vi "Auto-IR Logic.vi"(4 "Reset":bool, 6 "Upper Mag IR":T1, 7 "Rear Enter IR":T1) -> (0 "Finished":bool, 1 "Roller Output":dbl, 2 "Upper Mag IR Out":T1, 3 "Rear Enter IR Out":T1)   [LabVIEW 2011]
uses:
  <vilib>/Rock Robotics/WPI/DigitalInput/WPI_DigitalInputDevRef.ctl
  <vilib>/Rock Robotics/SystemInterfaces/DIO/FPGA_DIOChannel.ctl
  <vilib>/Rock Robotics/SystemInterfaces/Typedef/FPGA_TypedefDigitalModule.ctl
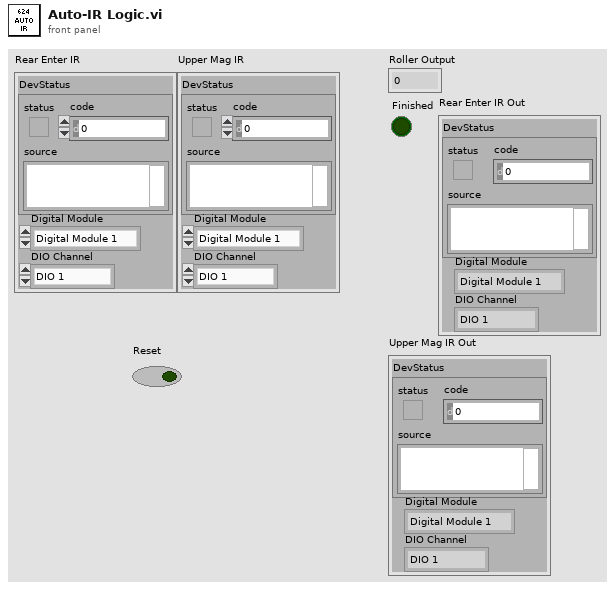
[diagram p1: front panel]
types:
  T1 = typedef "WPI_DigitalInputDevRef.ctl" = cluster{"DevStatus":errorcluster, "DIO Channel":T2, "Digital Module":T3}
  T2 = typedef "FPGA_DIOChannel.ctl" = enum8{"DIO 1", "DIO 2", "DIO 3", "DIO 4", "DIO 5", "DIO 6", "DIO 7", "DIO 8", "DIO 9", "DIO 10", "DIO 11", "DIO 12", "DIO 13", "DIO 14", "Invalid"}
  T3 = typedef "FPGA_TypedefDigitalModule.ctl" = enum16{"Digital Module 1", "Digital Module 2"}
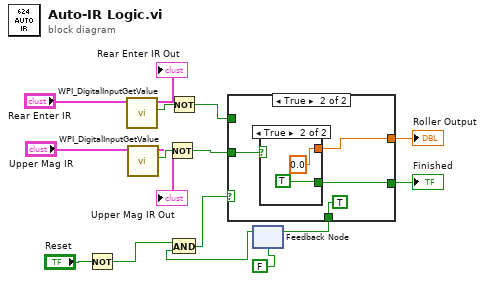
[diagram p0: block diagram]
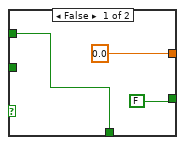
[diagram p2: hidden frame]
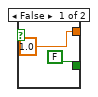
[diagram p3: hidden frame]
diagram:
  n1 = Not(x="Reset") -> (.not. x?=w5:bool)
  n2 = call <vilib>:"WPI_DigitalInputGetValue.vi"("DigitalInputDevRef"="Rear Enter IR") -> ("Value"=w16:bool, "DigitalInputDevRef"=→"Rear Enter IR Out":T1)  [unwired: 8 in, 1 out]
  n3 = call <vilib>:"WPI_DigitalInputGetValue.vi"("DigitalInputDevRef"="Upper Mag IR") -> ("Value"=w15:bool, "DigitalInputDevRef"=→"Upper Mag IR Out":T1)  [unwired: 8 in, 1 out]
  n4 = Not(x=w15) -> (.not. x?=w8:bool)
  n5 = Not(x=w16) -> (.not. x?=w13:bool)
  n6 = feedback #1(FALSE) -> (w6:bool)
  n7 = And(x=w5, y=w6) -> (x .and. y?=w7:bool)
  n8 = case shown="True" w7 {
    tunnel: [0.0 ("Output") w23] -> w4
    tunnel: [FALSE w22] -> w3
    tunnel: w8 -> [_ w21]
    tunnel: [w17 TRUE] -> w12
    tunnel: w13 -> [w17 _]
    frame False {
    }
    frame True {
      n9 = case shown="True" w21 {
        tunnel: [1.0 ("Output") 0.0 ("Output")] -> w23
        tunnel: [FALSE TRUE] -> w22
        frame False {
        }
        frame True {
        }
      }
    }
  }
  "Roller Output" <- w4
  "Finished" <- w3
  n10 = feedback-in #1(w12) -> ()
